vi "DMSS.construct_node_services.vi"(0 "domainName":string, 1 "processes":T1[](array[typedef]) {"restartMode" items=["UNKNOWN", "MANUAL", "ONCE", "ALWAYS", "KILL"]}, 2 "nodeName":string, 3 "CSSystems":string) -> (15 "taskList":string, 17 "CSSystems (out)":string)   [LabVIEW 2014, in "DMSServer.lvlib"]
doc: "constructs service strings using the process list (of a specific node)"
uses:
  DMSServer.lvlib
  DMSS.process_type.ctl
  DomainManagementUtils/DMSU.restart_mode.ctl
  DomainManagementUtils/DMSUtils.lvlib
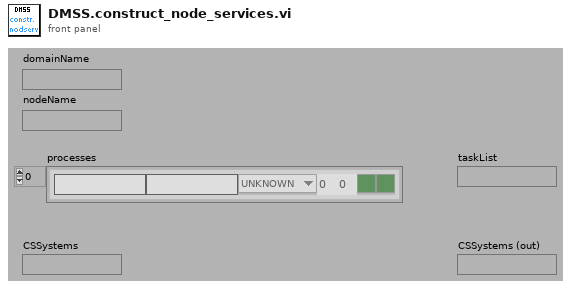
[diagram p1: front panel]
types:
  T1 = typedef "DMSServer.lvlib/DMSS.process_type.ctl" = cluster{"imageName":string, "argumentString":string, "restartMode":T2, "nOfRestart":i32, "resetRestartTimer":i32, "killOnExit":bool, "csSystem":bool}
  T2 = typedef "DMSUtils.lvlib/DMSU.restart_mode.ctl" = u16
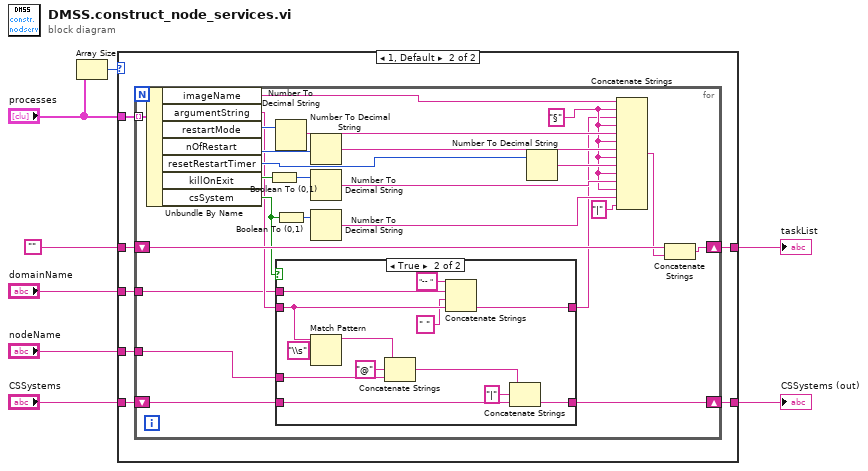
[diagram p0: block diagram]
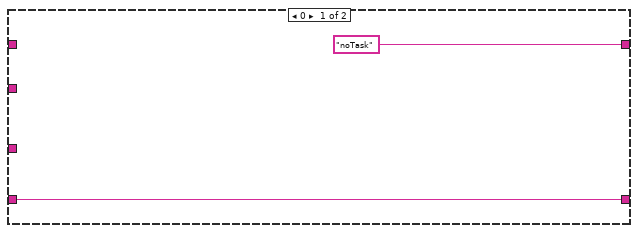
[diagram p2: hidden frame]
diagram:
  n1 = Array Size(array="processes") -> (size(s)=w1:i32)
  n2 = case shown="1, Default" w1 {
    tunnel: ["noTask" w17] -> w8
    tunnel: [w9 w16] -> w7
    tunnel: "CSSystems" -> [w9 w15]
    tunnel: "" ("Empty String Constant") -> [_ w14]
    tunnel: "nodeName" -> [_ w13]
    tunnel: "domainName" -> [_ w12]
    tunnel: "processes" -> [_ w11]
    frame 0 {
    }
    frame 1, Default {
      n3 = for {
        tunnel: w11 -> [w42] mode=indexing
        shift-right: [w29] -> w17
        shift-left: w14 -> [w28]
        shift-right: [w24] -> w16
        shift-left: w15 -> [w25]
        tunnel: w13 -> [w19]
        tunnel: w12 -> [w18]
        w23 = "§" ("string")
        n4 = Unbundle By Name(w42) -> ("imageName"=w21:string, "argumentString"=w22:string, "restartMode"=w41:T2, "nOfRestart"=w40:i32, "resetRestartTimer"=w36:i32, "killOnExit"=w35:bool, "csSystem"=w26:bool)
        n5 = Boolean To (0,1)(Boolean=w35) -> (0, 1=w34:i16)
        n6 = Number To Decimal String(number=w41) -> (decimal integer string=w39:string)  [unwired: 1 in]
        n7 = Boolean To (0,1)(Boolean=w26) -> (0, 1=w32:i16)
        n8 = case shown="True" w26 {
          tunnel: w22 -> [w43 w49]
          tunnel: w25 -> [w44 w56]
          tunnel: [w44 w55] -> w24
          tunnel: [w43 w46] -> w20
          tunnel: w19 -> [_ w51]
          tunnel: w18 -> [_ w48]
          frame False {
          }
          frame True {
            n9 = Match Pattern(string=w49, regular expression="\\s") -> (before substring=w53:string)  [unwired: 1 in, 3 out]
            n10 = Concatenate Strings(w53, "@" ("string"), w51) -> (w50:string)
            n11 = Concatenate Strings("-- " ("string"), w48, " " ("string"), w49) -> (w46:string)
            n12 = Concatenate Strings(w50, "|" ("string"), w56) -> (w55:string)
          }
        }
        n13 = Number To Decimal String(number=w40) -> (decimal integer string=w38:string)  [unwired: 1 in]
        n14 = Number To Decimal String(number=w34) -> (decimal integer string=w33:string)  [unwired: 1 in]
        n15 = Number To Decimal String(number=w32) -> (decimal integer string=w31:string)  [unwired: 1 in]
        n16 = Number To Decimal String(number=w36) -> (decimal integer string=w37:string)  [unwired: 1 in]
        n17 = Concatenate Strings(w21, w23, w20, w23, w39, w23, w38, w23, w37, w23, w33, w23, w31, "|" ("string")) -> (w27:string)
        n18 = Concatenate Strings(w28, w27) -> (w29:string)
      }
    }
  }
  "taskList" <- w8
  "CSSystems (out)" <- w7
